vi "Address.vi"(7 "报告类型":u16(ring)=1, 8 "错误簇输入":errorcluster, 9 "路径":path=path "C:/ report 3.doc", 10 "保存？":bool, 11 "报告输入":T1) -> (0 "错误簇输出":errorcluster, 3 "报告输出":T1)   [LabVIEW 2012]
uses:
  <vilib>/Utility/NIReport.llb/Generate Report Object Reference.ctl
  <vilib>/Utility/NIReport.llb/NI_report.lvclass
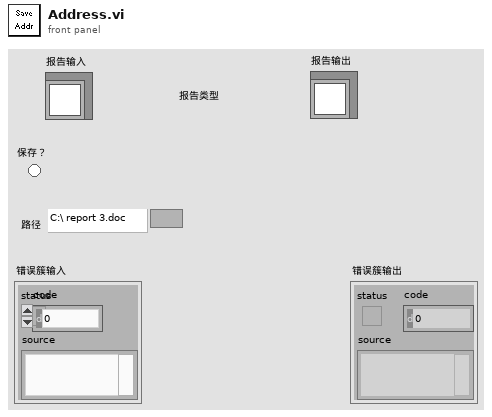
[diagram p1: front panel]
types:
  T1 = typedef "Generate Report Object Reference.ctl" = refnum<class "NI_report.lvclass">
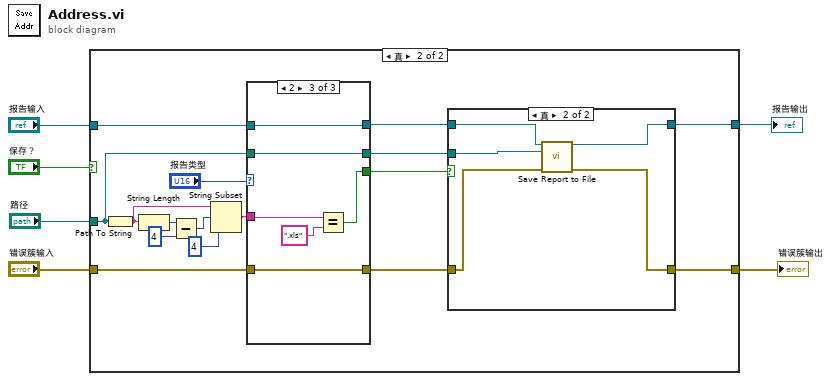
[diagram p0: block diagram]
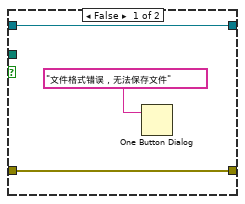
[diagram p3: hidden frame]
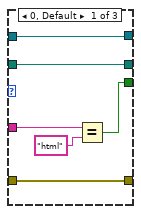
[diagram p4: hidden frame]
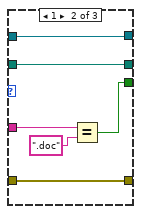
[diagram p5: hidden frame]
diagram:
  n1 = case shown="真" "保存？" {
    tunnel: "报告输入" -> [w8 w23]
    tunnel: "路径" -> [_ w9]
    tunnel: [w8 w13] -> w3
    tunnel: "错误簇输入" -> [w7 w16]
    tunnel: [w7 w11] -> w1
    frame False {
    }
    frame True {
      n2 = Path To String(path=w9) -> (string=w18:string)
      n3 = String Length(string=w18) -> (length=w19:i32)
      n4 = Subtract(x=w19, y=4) -> (x-y=w21:i32)
      n5 = String Subset(string=w18, offset (0)=w21, length (rest)=4 ("长度（剩余）")) -> (substring=w17:string)
      n6 = case shown="2" "报告类型" {
        tunnel: w23 -> [w35 w41 w47]
        tunnel: w17 -> [w37 w43 w49]
        tunnel: [w35 w41 w47] -> w12
        tunnel: w16 -> [w34 w40 w46]
        tunnel: [w36 w42 w48] -> w15
        tunnel: [w34 w40 w46] -> w14
        tunnel: [w33 w39 w45] -> w10
        tunnel: w9 -> [w33 w39 w45]
        frame 0, Default {
          n7 = Equal?(x=w37, y="html") -> (x = y?=w36:bool)
        }
        frame 1 {
          n8 = Equal?(x=w43, y=".doc") -> (x = y?=w42:bool)
        }
        frame 2 {
          n9 = Equal?(x=w49, y=".xls") -> (x = y?=w48:bool)
        }
      }
      n10 = case shown="真" w15 {
        tunnel: [w25 w32] -> w13
        tunnel: [w26 w31] -> w11
        tunnel: w14 -> [w26 w29]
        tunnel: w12 -> [w25 w30]
        tunnel: w10 -> [_ w28]
        frame False {
          n11 = One Button Dialog(message="文件格式错误，无法保存文件" ("消息")) -> ()  [unwired: 1 in, 1 out]
        }
        frame True {
          n12 = call-dynamic "Save Report to File.vi"("report in"=w30, "report file path"=w28, "error in (no error)"=w29) -> ("report out"=w32:T1, "error out"=w31:errorcluster)  [unwired: 11 in]
        }
      }
    }
  }
  "报告输出" <- w3
  "错误簇输出" <- w1
